vi "Read String Value (UTF-8 String).vi"(8 "error in":errorcluster, 11 "Control Ref":refnum<vi>) -> (0 "error out":errorcluster, 2 "UTF-8 String":refnum<class "UTF-8 String.lvclass">)   [LabVIEW 2020, in "G-Unicode.lvlib"]
doc: "Reads text from a control or indicator, converting between encodings as necessary. <b>UTF-8 String</b> will be a scalar value, 1D array, or 2D array depending on <b>Control Ref</b> type.\n\nThe control text output will be converted to UTF-8 from either UTF-16LE or ANSI, depending on the control's Interpret As Unicode property or text Byte Order Mark (BOM).\n\nSupported control/indicator types and their outputs:\n- String (scalar)\n- String Array (1D)\n- String Array (2D)\n- Ring Text (1D)\n- Tab Pages (1D)\n- Boolean Text (1D, 4 elements)\n- Table (2D)\n- Listbox (1D)\n- Multicolumn Listbox (2D)"
uses:
  G-Unicode.lvlib
  bfba3187-b22e-4285-8cc2-1816a803f974.vi
  Types/UTF-8 String/UTF-8 String.lvclass
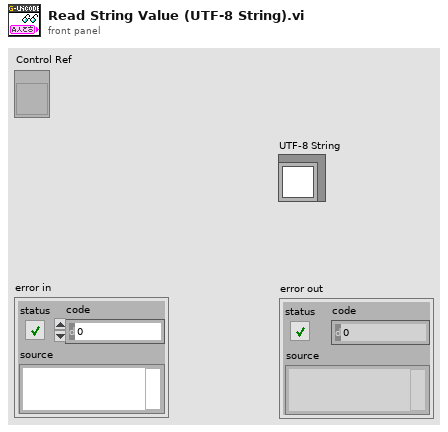
[diagram p1: front panel]
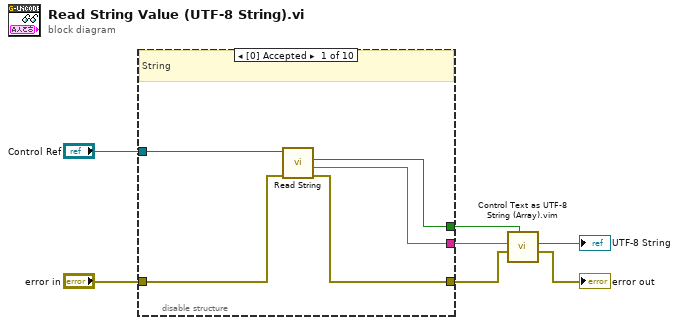
[diagram p0: block diagram]
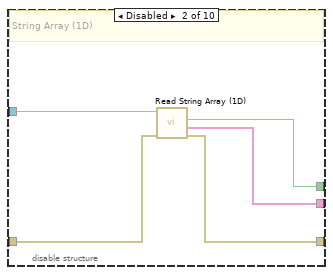
[diagram p2: hidden frame]
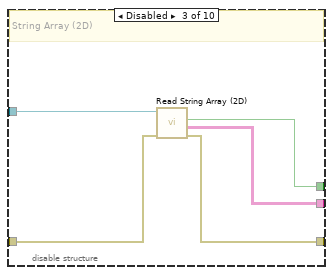
[diagram p3: hidden frame]
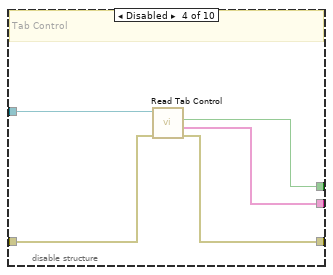
[diagram p4: hidden frame]
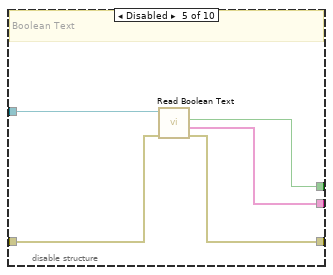
[diagram p5: hidden frame]
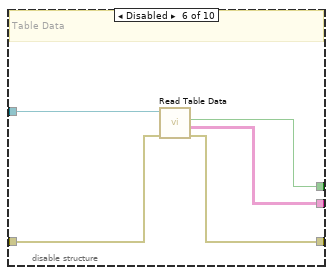
[diagram p6: hidden frame]
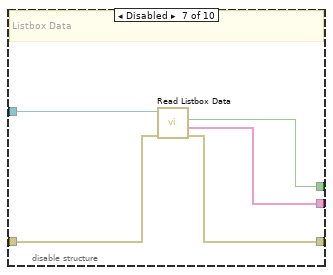
[diagram p7: hidden frame]
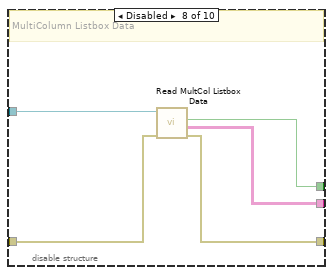
[diagram p8: hidden frame]
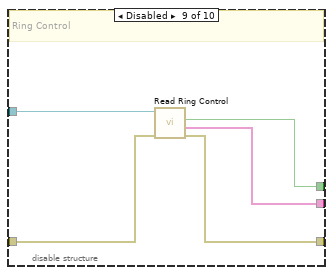
[diagram p9: hidden frame]
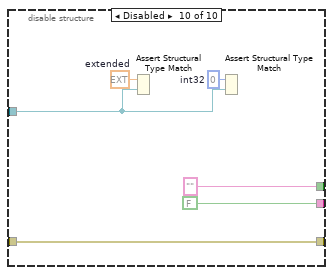
[diagram p10: hidden frame]
diagram:
  n1 = disable-structure "Type Specialization Structure" shown="[0] Accepted" {
    disable-tunnel: "Control Ref" -> [w12 w17 w22 w27 w32 w37 w42 w47 w52 w56]
    disable-tunnel: "error in" -> [w11 w16 w21 w26 w31 w36 w41 w46 w51 w55]
    disable-tunnel: [w9 w15 w19 w24 w29 w34 w39 w44 w49 "" ("Value")] -> w5
    disable-tunnel: [w10 w13 w20 w25 w30 w35 w40 w45 w50 w55] -> w2
    disable-tunnel: [w8 w14 w18 w23 w28 w33 w38 w43 w48 FALSE ("Text.InterpretAsUnicode")] -> w4
    frame Enabled {
      # "String"
      n2 = call "Read String.vi"("error in"=w11, "String Control Reference in"=w12) -> ("error out"=w10:errorcluster, "Value"=w8:string, "Interpret As Unicode"=w9:bool)  [unwired: 6 in, 1 out]
    }
    frame Disabled {
      # "String Array (1D)"
      n3 = call "Read String Array (1D).vi"("error in"=w16, "String Array (1D) Ref in"=w17) -> ("error out"=w13:errorcluster, "Value"=w14:string[], "Interpret As Unicode"=w15:bool)  [unwired: 6 in, 1 out]
    }
    frame Disabled {
      # "String Array (2D)"
      n4 = call "Read String Array (2D).vi"("error in"=w21, "String Array (2D) Ref in"=w22) -> ("error out"=w20:errorcluster, "Value"=w18:string[][], "Interpret As Unicode"=w19:bool)  [unwired: 6 in, 1 out]
    }
    frame Disabled {
      # "Tab Control"
      n5 = call "Read Tab Control.vi"("error in"=w26, "Tab Control in"=w27) -> ("error out"=w25:errorcluster, "Value"=w23:string[], "Interpret As Unicode"=w24:bool)  [unwired: 6 in, 1 out]
    }
    frame Disabled {
      # "Boolean Text"
      n6 = call "Read Boolean Text.vi"("error in"=w31, "Boolean Reference in"=w32) -> ("error out"=w30:errorcluster, "Value"=w28:string[], "Interpret As Unicode"=w29:bool)  [unwired: 6 in, 1 out]
    }
    frame Disabled {
      # "Table Data"
      n7 = call "Read Table Data.vi"("error in"=w36, "Table Ref in"=w37) -> ("error out"=w35:errorcluster, "Value"=w33:string[][], "Interpret As Unicode"=w34:bool)  [unwired: 6 in, 1 out]
    }
    frame Disabled {
      # "Listbox Data"
      n8 = call "Read Listbox Data.vi"("error in"=w41, "Listbox Ref in"=w42) -> ("error out"=w40:errorcluster, "Value"=w38:string[], "Interpret As Unicode"=w39:bool)  [unwired: 6 in, 1 out]
    }
    frame Disabled {
      # "MultiColumn Listbox Data"
      n9 = call "Read MultCol Listbox Data.vi"("error in"=w46, "Multicolumn Listbox Ref in"=w47) -> ("error out"=w45:errorcluster, "Value"=w43:string[][], "Interpret As Unicode"=w44:bool)  [unwired: 6 in, 1 out]
    }
    frame Disabled {
      # "Ring Control"
      n10 = call "Read Ring Control.vi"("error in"=w51, "Ring Control Ref in"=w52) -> ("error out"=w50:errorcluster, "Value"=w48:string[], "Interpret As Unicode"=w49:bool)  [unwired: 6 in, 1 out]
    }
    frame Disabled {
      w57 = 0  # int32
      w58 = ext 0.0  # extended
      n11 = Assert Structural Type Match(0:w56, 1:w58) -> ()
      n12 = Assert Structural Type Match(0:w56, 1:w57) -> ()
    }
  }
  n13 = call "Control Text as UTF-8 String (Array).vim"("Interpret As Unicode"=w5, "error in"=w2, "Control Text"=w4) -> ("error out"=→"error out":errorcluster, "UTF-8 String"=→"UTF-8 String":refnum<class "UTF-8 String.lvclass">)  [unwired: 7 in]
